vi "Accept Or Decline.vi"(6 "Additional Events":T1, 7 "timeout":i32=200, 8 "error in (no error)":errorcluster, 10 "MM Gui Updates In":refnum<queue>, 11 "MM Button Events In":refnum<notifier>) -> (0 "error out":errorcluster, 1 "Accepted or Declined":T2, 2 "MM Gui Updates Out":refnum<queue>, 3 "Button Events Out":refnum<notifier>)   [LabVIEW 2009]
uses:
  Mixed Mode Button Events Message.ctl
  Mixed Mode Button Events.ctl
  Mixed Mode Widget Button States.ctl
  Mixed Mode Control Type.ctl
  Mixed Mode Gui Update Msg.ctl
  Mixed Mode GUI Update Type.ctl
  Target.ctl
  Data Access Objects/Metadata/LBCB Number.ctl
  Accepted or Declined.ctl
  Monitor Button Events.ctl
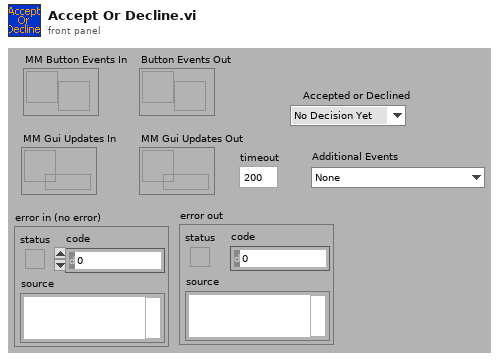
[diagram p1: front panel]
types:
  T1 = typedef "Monitor Button Events.ctl" = enum16{"None", "Running Event", "Connect NTCP Server Event"}
  T2 = typedef "Accepted or Declined.ctl" = enum16{"No Decision Yet", "Accepted", "Declined", "Abort"}
  T3 = typedef "Mixed Mode Gui Update Msg.ctl" = cluster{"MM GUI Update Type":T4, "Targets":T5[], "State":bool, "Step":string}
  T4 = typedef "Mixed Mode GUI Update Type.ctl" = enum16{"Nop", "Targets", "Accept.Blink", "Start.Blink", "TestStats", "Control.Enabled", "StartTestTimer", "RunInputFile", "NTCP Server"}
  T5 = typedef "Target.ctl" = cluster{"LBCB Number":T6, "DOF Vectors":enum16{" ", "Dx", "Dy", "Dz", "Rx", "Ry", "Rz", "Fx", "Fy", "Fz", "Mx", "My", "Mz"}, "Amount":dbl}
  T6 = typedef "LBCB Number.ctl" = enum16{"LBCB1", "LBCB2"}
  T7 = typedef "Mixed Mode Button Events Message.ctl" = cluster{"MM Control Events":T8, "Button States":T9}
  T8 = typedef "Mixed Mode Button Events.ctl" = enum16{"Propose.Accept", "Propose.Decline", "Execute.Start", "Execute.Stop", "TargetChange", "InputFile.Load", "InputFile.Reset", "InputFile.Pause", "InputFile.Run", "CartesianType.Changed", "NCTP.ConnectToServer", "Application.Stop", "Control.Enabled", "Control.Disabled", "ControlType.Changed", "Nop"}
  T9 = typedef "Mixed Mode Widget Button States.ctl" = cluster{"Auto-Start Enabled":bool, "Auto-Accept Enabled":bool, "Exit Requested":bool, "Mixed Mode Control Type":T10, "Input File Loaded":bool, "Input File Running":bool, "NTCP Server  On":bool}
  T10 = typedef "Mixed Mode Control Type.ctl" = enum32{"Manual", "Input File", "NTCP"}
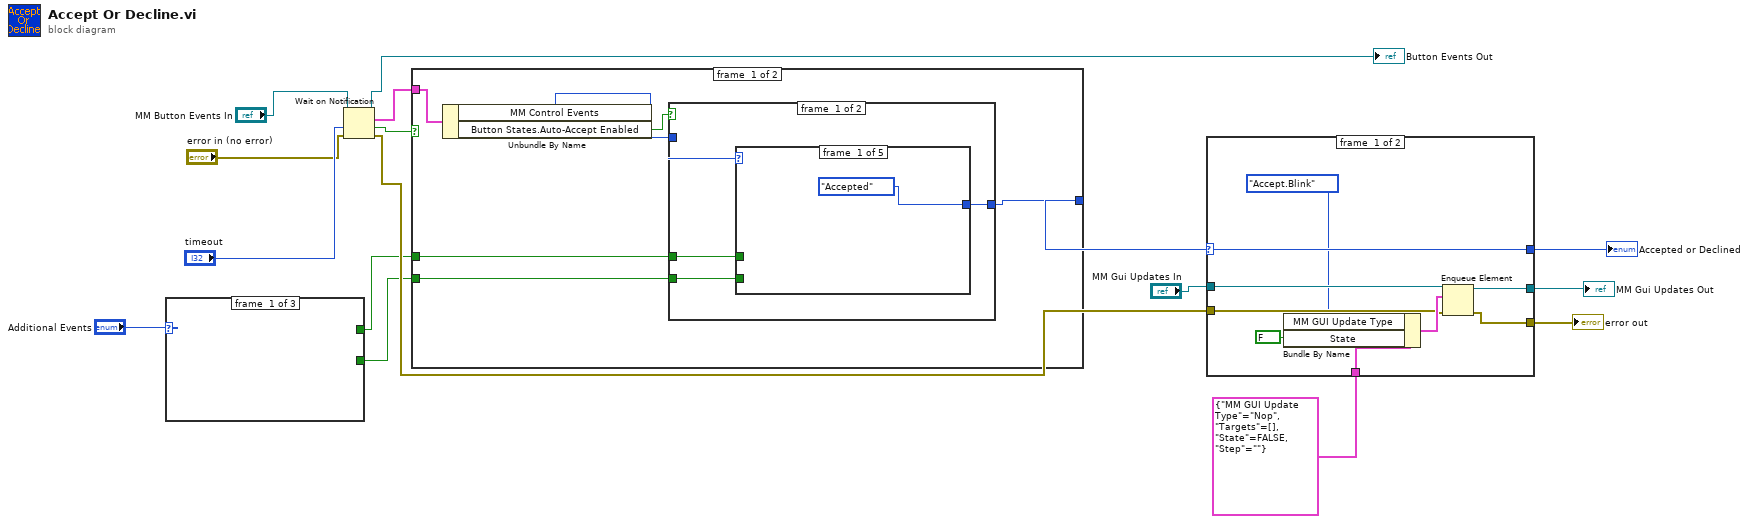
[diagram p0: block diagram]
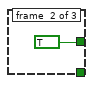
[diagram p2: hidden frame]
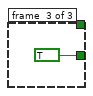
[diagram p3: hidden frame]
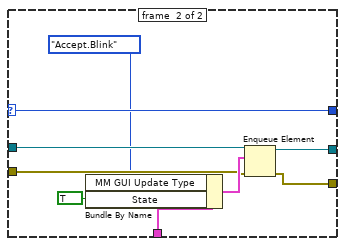
[diagram p4: hidden frame]
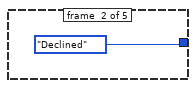
[diagram p5: hidden frame]
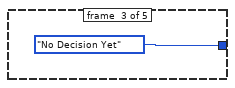
[diagram p6: hidden frame]
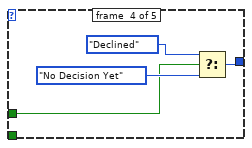
[diagram p7: hidden frame]
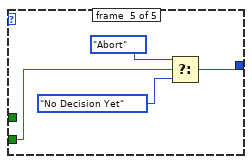
[diagram p8: hidden frame]
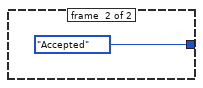
[diagram p9: hidden frame]
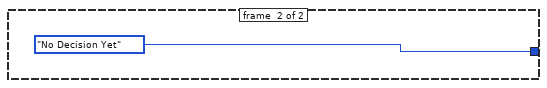
[diagram p10: hidden frame]
diagram:
  n1 = case shown="\"Connect NTCP Server Event\"" "Additional Events" {
    tunnel: [_ TRUE _] -> w2
    tunnel: [_ _ TRUE] -> w1
    frame #0 {
    }
    frame #1 {
    }
    frame #2 {
    }
  }
  n2 = Wait on Notification(notifier="MM Button Events In", timeout in ms (-1)="timeout", error in (no error)="error in (no error)") -> (notifier out=→"Button Events Out":refnum<notifier>, notification=w11:T7, timed out?=w12:bool, error out=w4:errorcluster)  [unwired: 1 in]
  n3 = case shown="False" w12 {
    tunnel: w11 -> [w24 _]
    tunnel: [w21 Accepted_or_Declined."No Decision Yet" ("Accepted or Declined")] -> w10
    tunnel: w2 -> [w20 _]
    tunnel: w1 -> [w19 _]
    frame #0 {
      n4 = Unbundle By Name(w24) -> ("MM Control Events"=w23:T8, "Button States.Auto-Accept Enabled"=w22:bool)
      n5 = case shown="False" w22 {
        tunnel: w23 -> [w28 _]
        tunnel: [w27 Accepted_or_Declined."Accepted" ("Accepted or Declined")] -> w21
        tunnel: w20 -> [w26 _]
        tunnel: w19 -> [w25 _]
        frame #0 {
          n6 = case shown="\"NCTP.ConnectToServer\"" w28 {
            tunnel: [Accepted_or_Declined."Accepted" ("Accepted or Declined") Accepted_or_Declined."Declined" ("Accepted or Declined") Accepted_or_Declined."No Decision Yet" ("Accepted or Declined") w35 w37] -> w27
            tunnel: w26 -> [_ _ _ w32 _]
            tunnel: w25 -> [_ _ _ _ w39]
            frame #0 {
            }
            frame #1 {
            }
            frame #2 {
            }
            frame #3 {
              n7 = Select(t=Accepted_or_Declined."Declined", s=w32, f=Accepted_or_Declined."No Decision Yet" ("Accepted or Declined")) -> (s? t:f=w35:T2)
            }
            frame #4 {
              n8 = Select(t=Accepted_or_Declined."Abort", s=w39, f=Accepted_or_Declined."No Decision Yet" ("Accepted or Declined")) -> (s? t:f=w37:T2)
            }
          }
        }
        frame #1 {
        }
      }
    }
    frame #1 {
    }
  }
  n9 = case shown="\"Accepted\", Default" w10 {
    selector: w10 -> [w50 w59]
    tunnel: [w50 w59] -> w9
    tunnel: "MM Gui Updates In" -> [w49 w58]
    tunnel: T3 {"MM GUI Update Type"=enum."Nop", "Targets"=[], "State"=FALSE, "Step"=""} ("element") -> [w48 w57]
    tunnel: [w46 w55] -> w6
    tunnel: [w45 w54] -> w5
    tunnel: w4 -> [w44 w53]
    frame #0 {
      n10 = Bundle By Name(cluster=w48, "MM GUI Update Type"=Mixed_Mode_GUI_Update_Type."Accept.Blink", "State"=FALSE) -> (w47:T3)
      n11 = Enqueue Element(queue=w49, element=w47, error in (no error)=w44) -> (queue out=w46:refnum<queue>, error out=w45:errorcluster)  [unwired: 1 in, 1 out]
    }
    frame #1 {
      n12 = Bundle By Name(cluster=w57, "MM GUI Update Type"=Mixed_Mode_GUI_Update_Type."Accept.Blink", "State"=TRUE) -> (w56:T3)
      n13 = Enqueue Element(queue=w58, element=w56, error in (no error)=w53) -> (queue out=w55:refnum<queue>, error out=w54:errorcluster)  [unwired: 1 in, 1 out]
    }
  }
  "Accepted or Declined" <- w9
  "MM Gui Updates Out" <- w6
  "error out" <- w5
